vi "Calcola compensaz scorr.vi"(6 "RPM nom":dbl, 9 "#poles":dbl, 10 "Fmax [Hz]":dbl, 11 "Fn [Hz]":dbl) -> (3 "%Fmax":dbl)   [LabVIEW 2019]
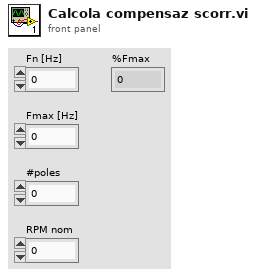
[diagram p1: front panel]
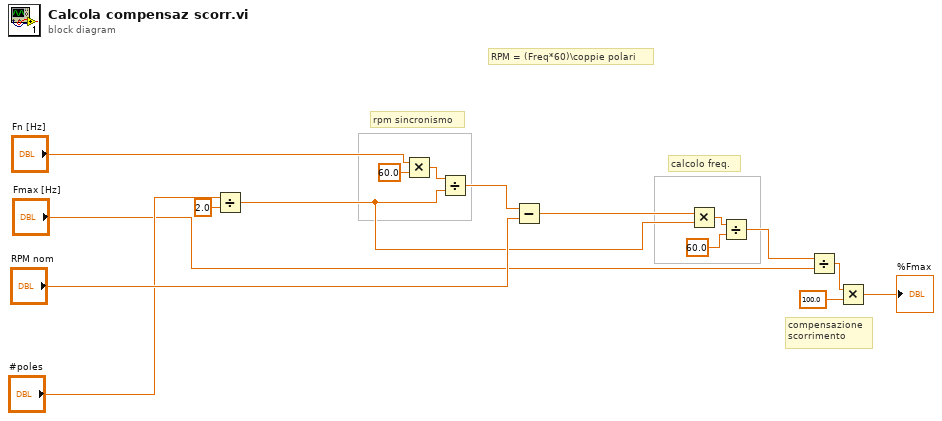
[diagram p0: block diagram]
diagram:
  # "RPM = (Freq*60)\\coppie polari"
  # "calcolo freq."
  # "compensazione\nscorrimento"
  # "rpm sincronismo"
  n1 = Divide(x="#poles", y=2.0) -> (x/y=w1:dbl)
  n2 = Multiply(x="Fn [Hz]", y=60.0) -> (x*y=w5:dbl)
  n3 = Divide(x=w5, y=w1) -> (x/y=w9:dbl)
  n4 = Subtract(x=w9, y="RPM nom") -> (x-y=w11:dbl)
  n5 = Multiply(x=w11, y=w1) -> (x*y=w12:dbl)
  n6 = Divide(x=w12, y=60.0) -> (x/y=w2:dbl)
  n7 = Divide(x=w2, y="Fmax [Hz]") -> (x/y=w14:dbl)
  n8 = Multiply(x=w14, y=100.0) -> (x*y=→"%Fmax":dbl)
